vi "Read Message.vi"(6 "error in":errorcluster, 8 "timeout ms (5000)":i32=5000, 9 "RawSocket Handler in":refnum<class "RawSocket TCP Handler.lvclass">) -> (0 "error out":errorcluster, 1 "Message data":u8[](array[numeric]), 2 "Message Type":T1, 3 "RawSocket Handler out":refnum<class "RawSocket TCP Handler.lvclass">)   [LabVIEW 2020, in "wamplv.lvlib" / "RawSocket TCP Handler.lvclass"]
uses:
  RawSocket TCP Handler.lvclass
  TypeDefs/Message Type.ctl
  RawSocket TCP Handler.lvclass/RawSocket TCP Handler.ctl
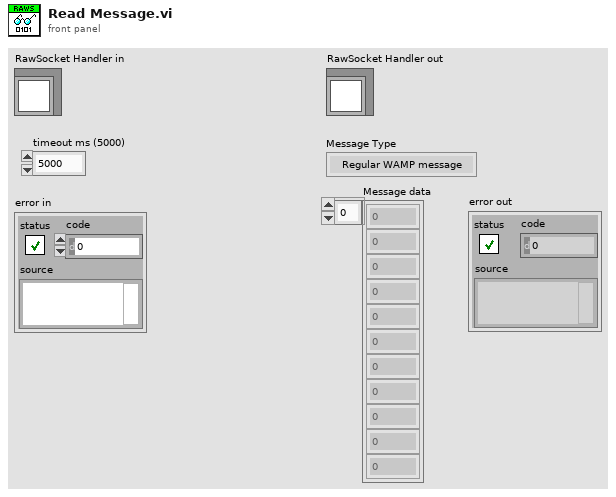
[diagram p1: front panel]
types:
  T1 = typedef "wamplv.lvlib/RawSocket TCP Handler.lvclass/Message Type.ctl" = enum8{"Regular WAMP message", "PING", "PONG"}
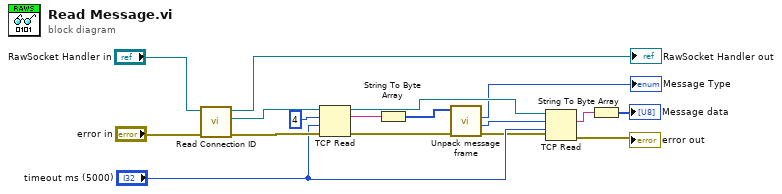
[diagram p0: block diagram]
diagram:
  n1 = call-dynamic "Read Connection ID.vi"("error in (no error)"="error in", "RawSocket Handler in"="RawSocket Handler in") -> ("error out"=w14:errorcluster, "Connection ID"=w13:refnum<k5>, "RawSocket Handler out"=→"RawSocket Handler out":refnum<class "RawSocket TCP Handler.lvclass">)  [unwired: 7 in]
  n2 = TCP Read(connection ID=w13, bytes to read=4, error in (no error)=w14, 9:"timeout ms (5000)") -> (connection ID out=w11:refnum<k5>, data out=w9:string, error out=w10:errorcluster)  [unwired: 1 in]
  n3 = String To Byte Array(string=w9) -> (unsigned byte array=w8:u8[])
  n4 = call "Unpack message frame.vi"("error in"=w10, "Message frame"=w8) -> ("error IO"=w6:errorcluster, "Size (bytes)"=w5:i32, "Message Type"=→"Message Type":T1)  [unwired: 7 in]
  n5 = TCP Read(connection ID=w11, bytes to read=w5, error in (no error)=w6, 9:"timeout ms (5000)") -> (data out=w2:string, error out=→"error out":errorcluster)  [unwired: 1 in, 1 out]
  n6 = String To Byte Array(string=w2) -> (unsigned byte array=→"Message data":u8[])
